vi "FindFirstMatch.vi"(8 "error in (no error)":errorcluster, 9 "xPath":string, 11 "NativeXML in":refnum<class "NativeXML.lvclass">) -> (0 "error out":errorcluster, 2 "NativeXML match":refnum<class "NativeXML.lvclass">, 3 "NativeXML out":refnum<class "NativeXML.lvclass">)   [LabVIEW 2009, in "Tools.lvlib" / "xml.lvlib" / "NativeXML.lvclass"]
uses:
  NativeXML.lvclass
  NativeXML.lvclass/NativeXML.ctl
  <vilib>/xml/NI_XML.lvlib
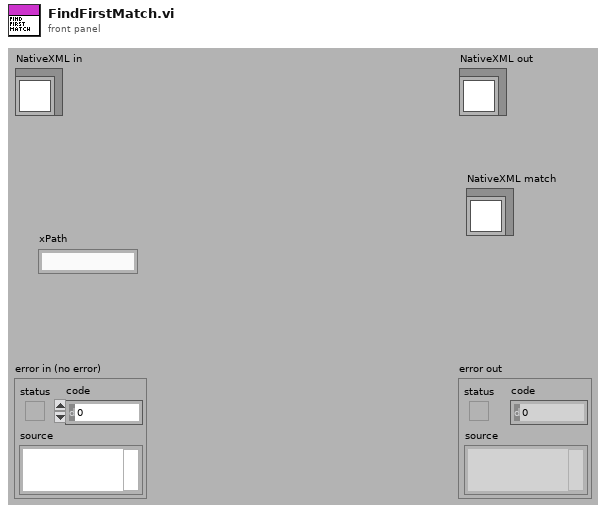
[diagram p1: front panel]
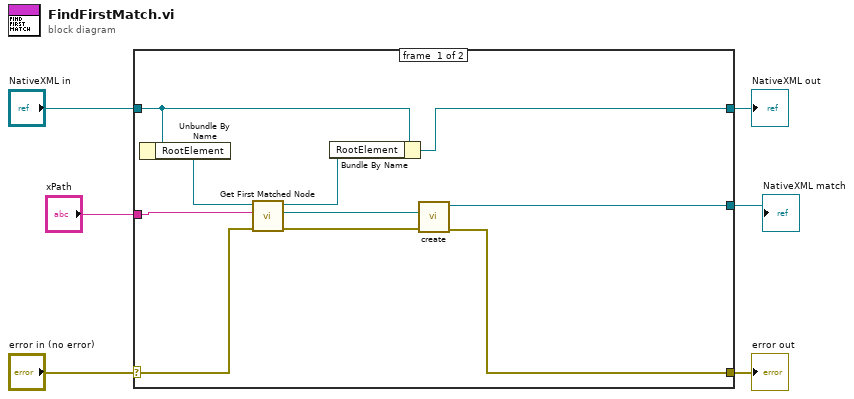
[diagram p0: block diagram]
diagram:
  n1 = case shown="No Error" "error in (no error)" {
    selector: "error in (no error)" -> [w9 w18]
    tunnel: [w8 w18] -> w5
    tunnel: [w12 w17] -> w3
    tunnel: "NativeXML in" -> [w13 w17]
    tunnel: "xPath" -> [w16 _]
    tunnel: [w7 _] -> w1
    frame #0 {
      n2 = Unbundle By Name(w13) -> ("RootElement"=w15:refnum<k20>)
      n3 = call <vilib>:"Get First Matched Node.vi"("error in (no error)"=w9, "XPath expression"=w16, "node in"=w15) -> ("error out"=w10:errorcluster, "node result"=w11:refnum<k20>, "node out"=w14:refnum<k20>)  [unwired: 6 in]
      n4 = Bundle By Name(cluster=w13, "RootElement"=w14) -> (w12:refnum<class "NativeXML.lvclass">)
      n5 = call "create.vi"("error in (no error)"=w10, "RootElement"=w11) -> ("error out"=w8:errorcluster, "NativeXML out"=w7:refnum<class "NativeXML.lvclass">)  [unwired: 8 in]
    }
    frame #1 {
    }
  }
  "error out" <- w5
  "NativeXML out" <- w3
  "NativeXML match" <- w1
